vi "Run Hashes.vi"() -> (3 "relative performance":cluster{i32[], dbl[]}[](graph)=[{[1, 10, 100, 500, 1000, 1500, 2000, 2500, 3500, 5000, 10000, 15000, 20000, 50000], [0.8857499997247942, 1.5753799999401963, 0.8115099999986342, 0.3211510000000999, 0.2594943249996504, 0.22179791666652213, 0.21387263750034435, 0.2069699600000604, 0.20111649285692174, 0.20029643000007127, 0.1994950074999906, 0.198307363333303, 0.19667207500001496, 0.196204838499998]}, {[1, 10, 100, 500, 1000], [50.52650000016001, 2.9727324999839766, 5.995129999996607, 5.990132599999924, 6.039437249999992]}])   [LabVIEW 2019, in "Redis Client Examples.lvlib"]
uses:
  Redis Client Examples.lvlib
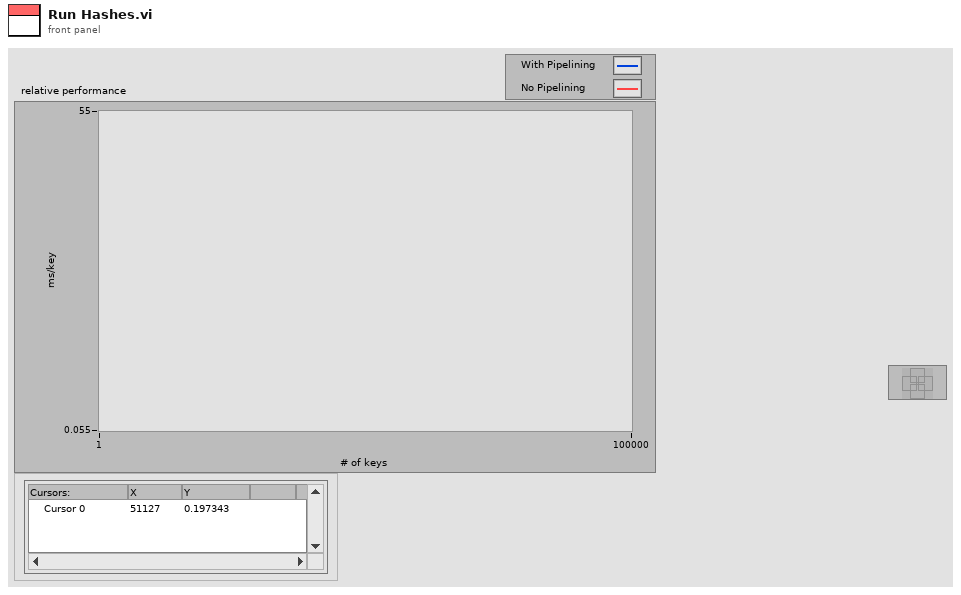
[diagram p1: front panel]
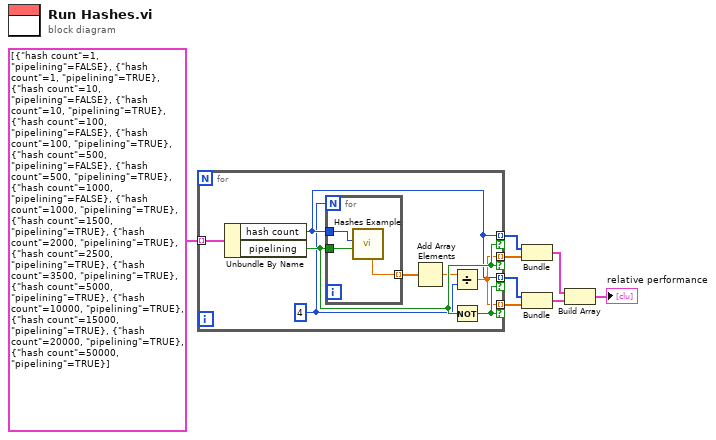
[diagram p0: block diagram]
diagram:
  n1 = for {
    tunnel: cluster{"hash count":i32, "pipelining":bool}[] [{"hash count"=1, "pipelining"=FALSE}, {"hash count"=1, "pipelining"=TRUE}, {"hash count"=10, "pipelining"=FALSE}, {"hash count"=10, "pipelining"=TRUE}, {"hash count"=100, "pipelining"=FALSE}, {"hash count"=100, "pipelining"=TRUE}, {"hash count"=500, "pipelining"=FALSE}, {"hash count"=500, "pipelining"=TRUE}, {"hash count"=1000, "pipelining"=FALSE}, {"hash count"=1000, "pipelining"=TRUE}, {"hash count"=1500, "pipelining"=TRUE}, {"hash count"=2000, "pipelining"=TRUE}, {"hash count"=2500, "pipelining"=TRUE}, {"hash count"=3500, "pipelining"=TRUE}, {"hash count"=5000, "pipelining"=TRUE}, {"hash count"=10000, "pipelining"=TRUE}, {"hash count"=15000, "pipelining"=TRUE}, {"hash count"=20000, "pipelining"=TRUE}, {"hash count"=50000, "pipelining"=TRUE}] -> [w16] mode=indexing
    tunnel: [w14] -> w7 mode=indexing if=w15
    tunnel: [w10] -> w6 mode=indexing if=w15
    tunnel: [w14] -> w5 mode=indexing if=w13
    tunnel: [w10] -> w4 mode=indexing if=w13
    w11 = 4
    n2 = Unbundle By Name(w16) -> ("hash count"=w14:i32, "pipelining"=w15:bool)
    n3 = for {
      N: w11 -> [_]
      tunnel: w15 -> [w19]
      tunnel: w14 -> [w18]
      tunnel: [w17] -> w12 mode=indexing
      n4 = call "Hashes Example.vi"("pipelining enabled?"=w19, "# of keys to test"=w18) -> ("execution time (ms/key)"=w17:dbl)  [unwired: 5 in, 4 out]
    }
    n5 = Add Array Elements(numeric array=w12) -> (sum=w9:dbl)
    n6 = Divide(x=w9, y=w11) -> (x/y=w10:dbl)
    n7 = Not(x=w15) -> (.not. x?=w13:bool)
  }
  n8 = Bundle(w7, w6) -> (w3:cluster{i32[], dbl[]})  [unwired: 1 in]
  n9 = Bundle(w5, w4) -> (w2:cluster{i32[], dbl[]})  [unwired: 1 in]
  n10 = Build Array(w3, w2) -> (→"relative performance":cluster{i32[], dbl[]}[])
